vi "Creat.vi"(8 "错误输入（无错误）":errorcluster, 11 "名称":string) -> (0 "错误输出":errorcluster, 3 "队列输出":refnum<queue>)   [LabVIEW 2020]
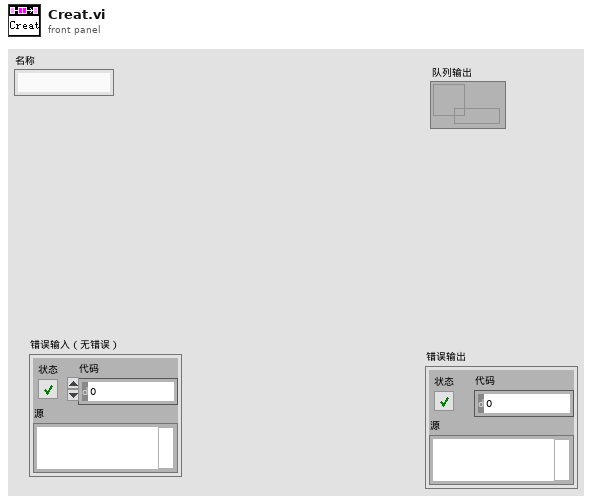
[diagram p1: front panel]
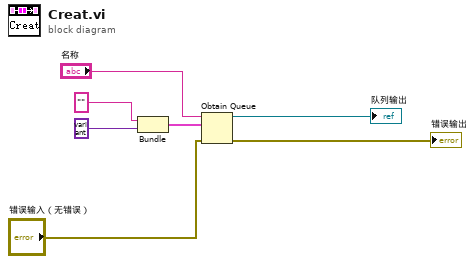
[diagram p0: block diagram]
diagram:
  n1 = Bundle("指令"="", "数据"=variant) -> (w5:cluster{"指令":string, "数据":variant})  [unwired: 1 in]
  n2 = Obtain Queue(name (unnamed)="名称", element data type=w5, error in (no error)="错误输入（无错误）") -> (queue out=→"队列输出":refnum<queue>, error out=→"错误输出":errorcluster)  [unwired: 2 in, 1 out]
